vi "CSV Series Reader.vi"(8 "error in":errorcluster, 11 "Filenames":string[](array[string])) -> (0 "error out":errorcluster, 3 "Data Series":T1)   [LabVIEW 2018, in "CSV Series Read.lvlib"]
uses:
  CSV Series Read.lvlib
  Data Series.ctl
  State Series.ctl
  E series.ctl
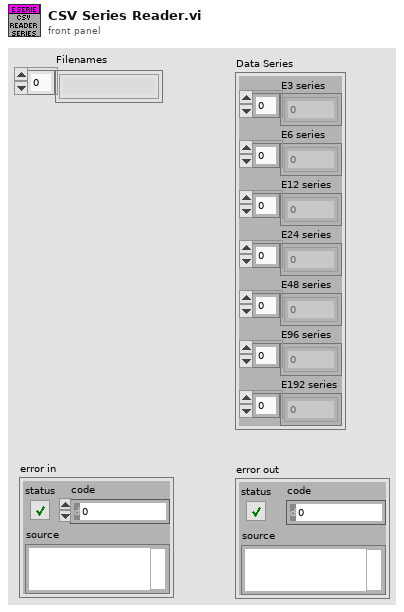
[diagram p1: front panel]
types:
  T1 = typedef "CSV Series Read.lvlib/Data Series.ctl" = cluster{"E3 series":u16[], "E6 series":u16[], "E12 series":u16[], "E24 series":u16[], "E48 series":u16[], "E96 series":u16[], "E192 series":u16[]}
  T2 = typedef "CSV Series Read.lvlib/State Series.ctl" = enum16{"Initialize", "E series 3", "E series 6", "E series 12", "E series 24", "E series 48", "E series 96", "E series 192", "Error", "Shutdown"}
  T3 = typedef "CSV Series Read.lvlib/E series.ctl" = enum16{"E series 3", "E series 6", "E series 12", "E series 24", "E series 48", "E series 96", "E series 192"}
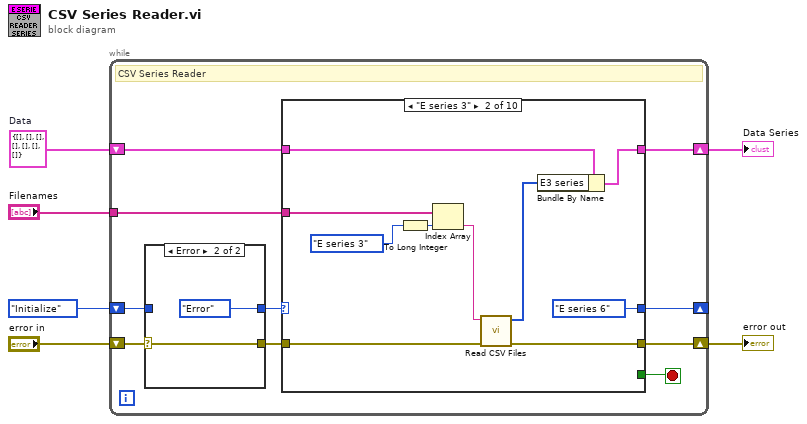
[diagram p0: block diagram]
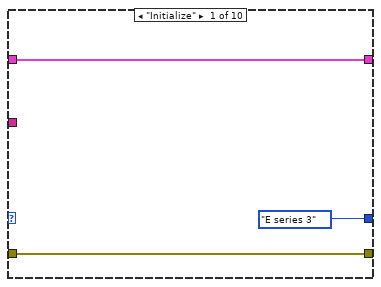
[diagram p3: hidden frame]
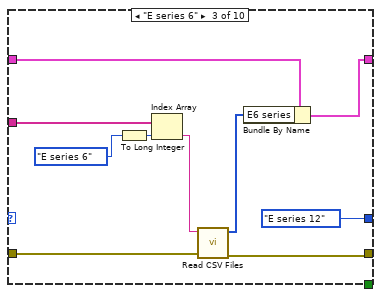
[diagram p4: hidden frame]
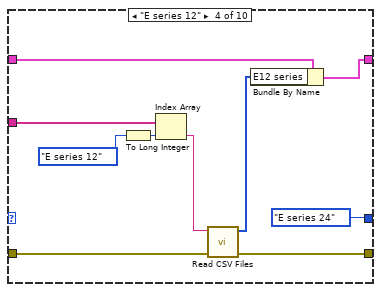
[diagram p5: hidden frame]
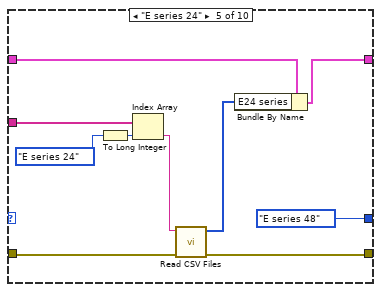
[diagram p6: hidden frame]
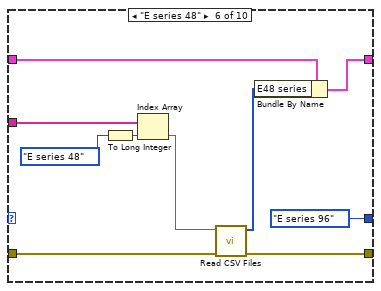
[diagram p7: hidden frame]
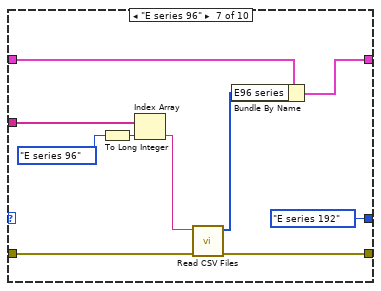
[diagram p8: hidden frame]
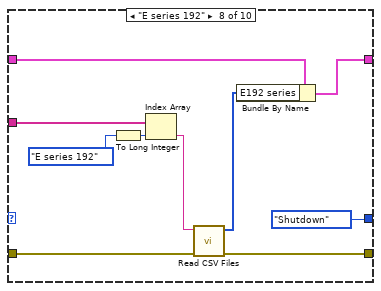
[diagram p9: hidden frame]
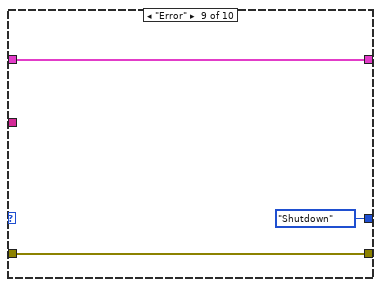
[diagram p10: hidden frame]
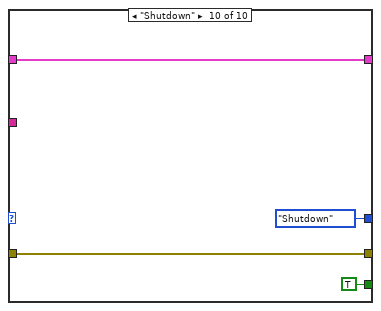
[diagram p11: hidden frame]
diagram:
  w3 = T1 {"E3 series"=[], "E6 series"=[], "E12 series"=[], "E24 series"=[], "E48 series"=[], "E96 series"=[], "E192 series"=[]}  # Data
  n1 = while {
    shift-right: [w11] -> _
    shift-left: State_Series."Initialize" ("Enum") -> [w14]
    shift-right: [w13] -> w5
    shift-left: "error in" -> [w12]
    shift-right: [w8] -> w2
    shift-left: w3 -> [w10]
    tunnel: "Filenames" -> [w7]
    stop <- w9 stop-if-true
    # "CSV Series Reader"
    n2 = case shown="Error" w12 {
      selector: w12 -> [w17 w20]
      tunnel: w14 -> [w18 _]
      tunnel: [w18 State_Series."Error" ("Enum")] -> w16
      tunnel: [w17 w20] -> w15
      frame No Error {
      }
      frame Error {
      }
    }
    n3 = case shown="\"E series 3\"" w16 {
      tunnel: w15 -> [w23 w29 w39 w52 w60 w68 w82 w89 w96 w100]
      tunnel: [w23 w28 w38 w51 w59 w69 w81 w88 w96 w100] -> w13
      tunnel: [State_Series."E series 3" ("Enum") State_Series."E series 6" ("Enum") State_Series."E series 12" ("Enum") State_Series."E series 24" ("Enum") State_Series."E series 48" ("Enum") State_Series."E series 96" ("Enum") State_Series."E series 192" ("Enum") State_Series."Shutdown" ("Enum") State_Series."Shutdown" ("Enum") State_Series."Shutdown" ("Enum")] -> w11
      tunnel: w10 -> [w21 w32 w42 w48 w62 w72 w79 w90 w95 w97]
      tunnel: [w21 w31 w40 w49 w61 w71 w80 w91 w95 w97] -> w8
      tunnel: [_ _ _ _ _ _ _ _ _ TRUE] -> w9
      tunnel: w7 -> [_ w27 w35 w45 w55 w65 w75 w84 _ _]
      frame "Initialize" {
      }
      frame "E series 3" {
        n4 = To Long Integer(number=E_series."E series 3") -> (32bit integer=w24:i32)
        n5 = Index Array(array=w27, index=w24) -> (element=w26:string)
        n6 = call "Read CSV Files.vi"("error in (no error)"=w29, "Series file name"=w26) -> ("error out"=w28:errorcluster, "Series"=w33:u16[])  [unwired: 8 in]
        n7 = Bundle By Name(cluster=w32, "E3 series"=w33) -> (w31:T1)
      }
      frame "E series 6" {
        n8 = To Long Integer(number=E_series."E series 6") -> (32bit integer=w36:i32)
        n9 = Index Array(array=w35, index=w36) -> (element=w34:string)
        n10 = call "Read CSV Files.vi"("error in (no error)"=w39, "Series file name"=w34) -> ("error out"=w38:errorcluster, "Series"=w43:u16[])  [unwired: 8 in]
        n11 = Bundle By Name(cluster=w42, "E6 series"=w43) -> (w40:T1)
      }
      frame "E series 12" {
        n12 = To Long Integer(number=E_series."E series 12") -> (32bit integer=w46:i32)
        n13 = Index Array(array=w45, index=w46) -> (element=w44:string)
        n14 = call "Read CSV Files.vi"("error in (no error)"=w52, "Series file name"=w44) -> ("error out"=w51:errorcluster, "Series"=w53:u16[])  [unwired: 8 in]
        n15 = Bundle By Name(cluster=w48, "E12 series"=w53) -> (w49:T1)
      }
      frame "E series 24" {
        n16 = To Long Integer(number=E_series."E series 24") -> (32bit integer=w56:i32)
        n17 = Index Array(array=w55, index=w56) -> (element=w54:string)
        n18 = call "Read CSV Files.vi"("error in (no error)"=w60, "Series file name"=w54) -> ("error out"=w59:errorcluster, "Series"=w63:u16[])  [unwired: 8 in]
        n19 = Bundle By Name(cluster=w62, "E24 series"=w63) -> (w61:T1)
      }
      frame "E series 48" {
        n20 = To Long Integer(number=E_series."E series 48") -> (32bit integer=w66:i32)
        n21 = Index Array(array=w65, index=w66) -> (element=w64:string)
        n22 = call "Read CSV Files.vi"("error in (no error)"=w68, "Series file name"=w64) -> ("error out"=w69:errorcluster, "Series"=w73:u16[])  [unwired: 8 in]
        n23 = Bundle By Name(cluster=w72, "E48 series"=w73) -> (w71:T1)
      }
      frame "E series 96" {
        n24 = To Long Integer(number=E_series."E series 96") -> (32bit integer=w76:i32)
        n25 = Index Array(array=w75, index=w76) -> (element=w74:string)
        n26 = call "Read CSV Files.vi"("error in (no error)"=w82, "Series file name"=w74) -> ("error out"=w81:errorcluster, "Series"=w83:u16[])  [unwired: 8 in]
        n27 = Bundle By Name(cluster=w79, "E96 series"=w83) -> (w80:T1)
      }
      frame "E series 192" {
        n28 = To Long Integer(number=E_series."E series 192") -> (32bit integer=w86:i32)
        n29 = Index Array(array=w84, index=w86) -> (element=w85:string)
        n30 = call "Read CSV Files.vi"("error in (no error)"=w89, "Series file name"=w85) -> ("error out"=w88:errorcluster, "Series"=w93:u16[])  [unwired: 8 in]
        n31 = Bundle By Name(cluster=w90, "E192 series"=w93) -> (w91:T1)
      }
      frame "Error" {
      }
      frame "Shutdown" {
      }
    }
  }
  "error out" <- w5
  "Data Series" <- w2
